vi "Statistical measure - basics - 3.vi"(5 "Data measured":dbl[](array[numeric]), 9 "Data reference":dbl[](array[numeric])) -> (3 "x != y?":bool, 8 "Statistcs":T1 {"mean meas" format="%.10f"; "min meas" format="%.10f"; "max meas" format="%.10f"; "mean dev" format="%.10f"; "min dev" format="%.10f"; "max dev" format="%.10f"; "mean ref" format="%.10f"; "min ref" format="%.10f"; "max ref" format="%.10f"})   [LabVIEW 2019]
panel:
  # "Statistical Measure - Basics - 3"
  # "array size"
  # "Deviaton"
  # "Measured"
  # "Reference"
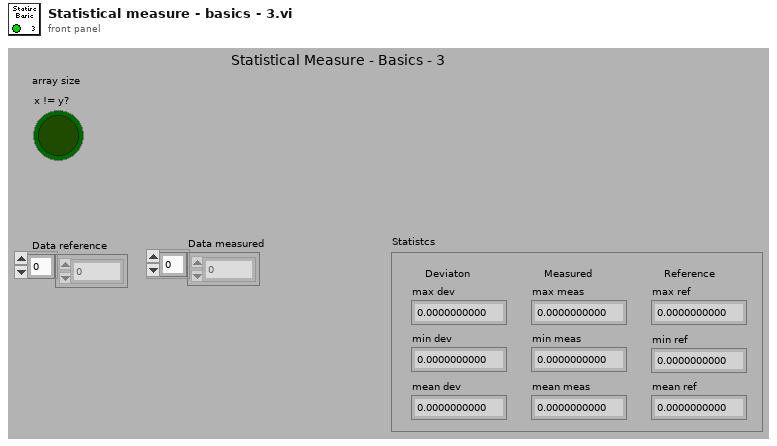
[diagram p1: front panel]
types:
  T1 = cluster{"max ref":dbl, "min ref":dbl, "mean ref":dbl, "max dev":dbl, "min dev":dbl, "mean dev":dbl, "max meas":dbl, "min meas":dbl, "mean meas":dbl}
  T2 = cluster{dbl, dbl, dbl, dbl, dbl, dbl, dbl, dbl, dbl}
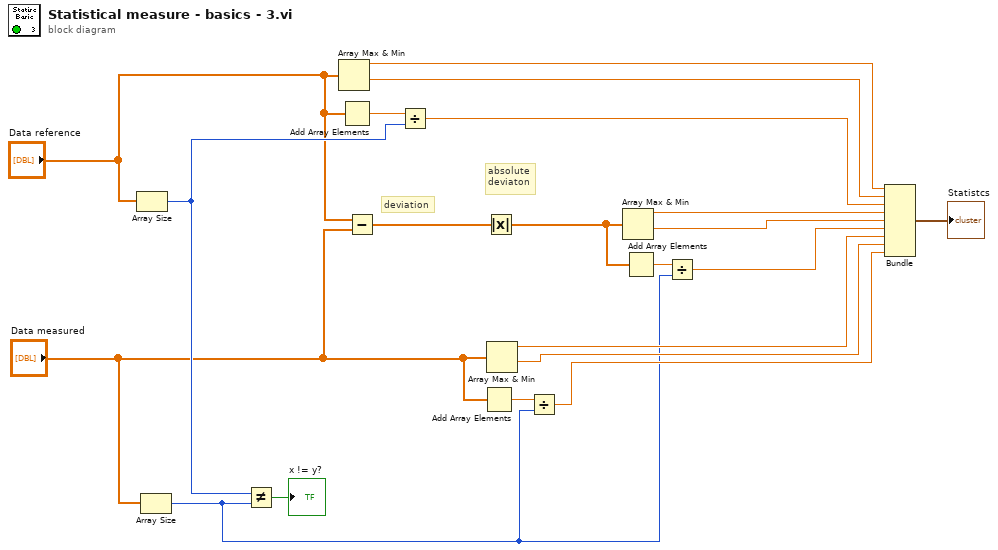
[diagram p0: block diagram]
diagram:
  # "absolute\ndeviaton"
  # "deviation"
  n1 = Array Size(array="Data reference") -> (size(s)=w19:i32)
  n2 = Array Size(array="Data measured") -> (size(s)=w10:i32)
  n3 = Not Equal?(x=w19, y=w10) -> (x != y?=→"x != y?":bool)
  n4 = Array Max & Min(array="Data reference") -> (max value=w6:dbl, min value=w5:dbl)  [unwired: 2 out]
  n5 = Add Array Elements(numeric array="Data reference") -> (sum=w3:dbl)
  n6 = Subtract(x="Data reference", y="Data measured") -> (x-y=w13:dbl[])
  n7 = Divide(x=w3, y=w19) -> (x/y=w4:dbl)
  n8 = Add Array Elements(numeric array="Data measured") -> (sum=w2:dbl)
  n9 = Absolute Value(x=w13) -> (abs(x)=w11:dbl[])
  n10 = Array Max & Min(array="Data measured") -> (max value=w17:dbl, min value=w16:dbl)  [unwired: 2 out]
  n11 = Divide(x=w2, y=w10) -> (x/y=w15:dbl)
  n12 = Array Max & Min(array=w11) -> (max value=w9:dbl, min value=w8:dbl)  [unwired: 2 out]
  n13 = Add Array Elements(numeric array=w11) -> (sum=w1:dbl)
  n14 = Divide(x=w1, y=w10) -> (x/y=w7:dbl)
  n15 = Bundle(w6, w5, w4, w9, w8, w7, w17, w16, w15) -> (→"Statistcs":T2)  [unwired: 1 in]
